vi "Test Sweep Manager.vi"(8 "error in (no error)":errorcluster, 11 "Lockin.DAQ in":refnum<class "Instrument.DAQ.lvclass">) -> (0 "error out":errorcluster, 3 "Lockin.DAQ out":refnum<class "Instrument.DAQ.lvclass">)   [LabVIEW 2019, in "Instrument.Lockin.lvlib" / "Instrument.DAQ.lvclass"]
uses:
  Instrument.DAQ.lvclass
  Typedefs/AO.Channel--Cluster--Array.ctl
  Typedefs/AO.Channel--Cluster.ctl
  Typedefs/AO.Channel.Function--Enum.ctl
  Typedefs/DAQ.Sampling.Sampling--Cluster.ctl
  Typedefs/Sweep.Configuration--Cluster.ctl
  Typedefs/Sweep.Channel--Cluster--Array.ctl
  Typedefs/Sweep.Channel--Cluster.ctl
  Typedefs/Sweep.Pattern--Enum.ctl
  Instrument.DAQ.lvclass/Instrument.DAQ.ctl
  <vilib>/Analysis/2dsp.llb/Decimate (single shot, DBL).vi
  <vilib>/Analysis/NI_AALPro.lvlib
  Instrument.Lockin/Instrument.Lockin.lvclass
panel:
  out "Waveform Graph 2":dbl[][](graph)
  in  "Sweep Pattern":cluster{"Channel":u16, "Sweep Pattern":dbl[]}[](array[cluster])=[{"Channel"=0, "Sweep Pattern"=[]}] {"Sweep Pattern" format="%#_3p"; "Channel" min=1 max=128}
  in  "milliseconds to wait":u32=1000
  out "Updates":i32
  out "Update":i32
  out "Waveform Graph":waveform(dbl)[](graph)
  in  "Configuration.Sweep":T1 {"Channels"."Table" format="%#_1f"; "Channels"."Channel" min=1 max=128; "Channels"."Start" format="%#_6p"; "Channels"."End" format="%#_6p"}
  in  "sampling":T5={"Fs"=204789.0, "#s"=15753} {"Fs" format="%#_13g"}
  in  "stop":bool
  in  "AO Channels":T6=[{"Enable?"=FALSE, "Channel"=0, "Amplitude"=0.0, "Offset"=0.0, "Frequency"=0.1, "Phase"=0.0, "Function"=enum."Sine", "Sweeping?"=FALSE}] {"Phase" format="%.3g"; "Frequency" min=0.0001 max=10000.0 format="%.3g"; "Offset" format="%.3p"; "Amplitude" min=0.0 max=10.0 format="%.3p"}
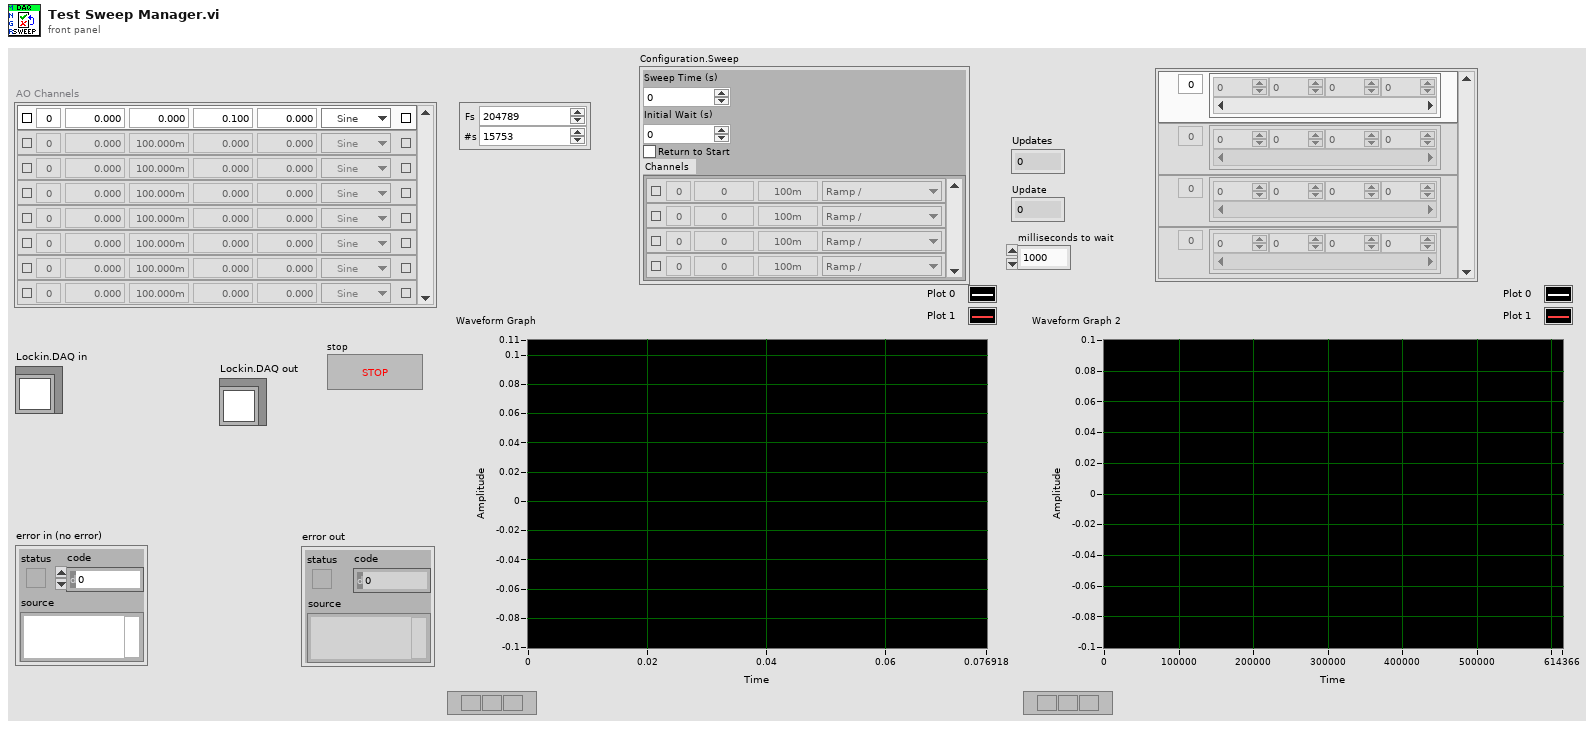
[diagram p1: front panel]
types:
  T1 = typedef "Instrument.Lockin.lvlib/Instrument.DAQ.lvclass/Sweep.Configuration--Cluster.ctl" = cluster{"Sweep Time (s)":dbl, "Initial Wait (s)":dbl, "Return to Start":bool, "Channels":T2}
  T2 = typedef "Instrument.Lockin.lvlib/Instrument.DAQ.lvclass/Sweep.Channel--Cluster--Array.ctl" = T3[]
  T3 = typedef "Instrument.Lockin.lvlib/Instrument.DAQ.lvclass/Sweep.Channel--Cluster.ctl" = cluster{"Enable?":bool, "Channel":u16, "Start":dbl, "End":dbl, "Pattern":T4, "Table":dbl[]}
  T4 = typedef "Instrument.Lockin.lvlib/Instrument.DAQ.lvclass/Sweep.Pattern--Enum.ctl" = enum16{"Ramp /", "Ramp /\\", "Smooth Ramp _/", "Smooth Ramp _/\\_", "Table"}
  T5 = typedef "Instrument.Lockin.lvlib/Instrument.DAQ.lvclass/DAQ.Sampling.Sampling--Cluster.ctl" = cluster{"Fs":dbl, "#s":i32}
  T6 = typedef "Instrument.Lockin.lvlib/Instrument.DAQ.lvclass/AO.Channel--Cluster--Array.ctl" = T7[]
  T7 = typedef "Instrument.Lockin.lvlib/Instrument.DAQ.lvclass/AO.Channel--Cluster.ctl" = cluster{"Enable?":bool, "Channel":i32, "Amplitude":dbl, "Offset":dbl, "Frequency":dbl, "Phase":dbl, "Function":T8, "Sweeping?":bool}
  T8 = typedef "Instrument.Lockin.lvlib/Instrument.DAQ.lvclass/AO.Channel.Function--Enum.ctl" = enum16{"Sine", "Triangle", "Square"}
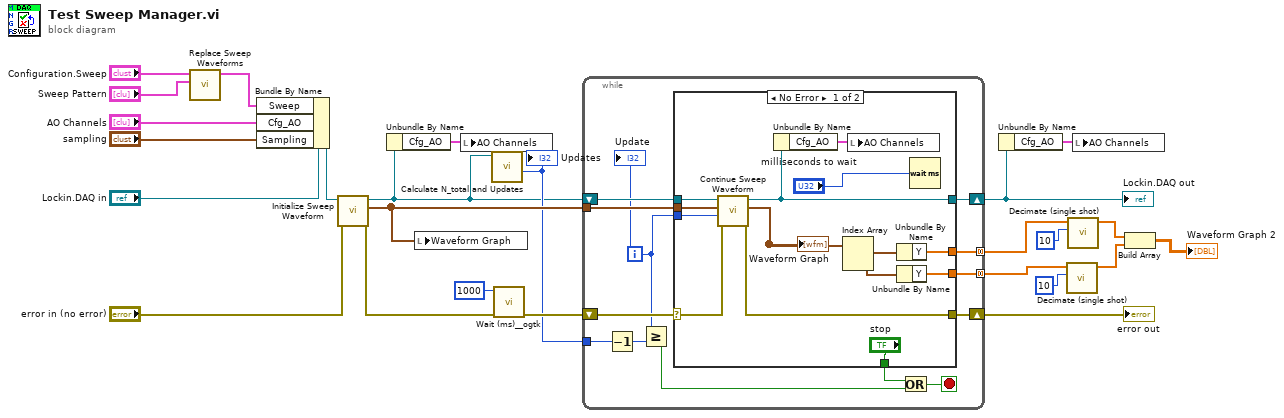
[diagram p0: block diagram]
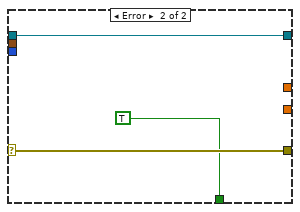
[diagram p2: hidden frame]
diagram:
  n1 = call "Replace Sweep Waveforms.vi"("Channels New"="Sweep Pattern", "Sweep in"="Configuration.Sweep") -> ("Sweep out"=w11:T1)  [unwired: 9 in]
  n2 = Bundle By Name(cluster="Lockin.DAQ in", "Sweep"=w11, "Cfg_AO"="AO Channels", "Sampling"="sampling") -> (w20:refnum<class "Instrument.DAQ.lvclass">)
  n3 = call "Initialize Sweep Waveform.vi"("error in (no error)"="error in (no error)", "Instrument.DAQ in"=w20) -> ("error out"=w15:errorcluster, "Waveforms"=w19:waveform(dbl)[], "Instrument.DAQ out"=w4:refnum<class "Instrument.DAQ.lvclass">)  [unwired: 7 in]
  n4 = Unbundle By Name(w4) -> ("Cfg_AO"=w3:T6)
  n5 = local write "Waveform Graph"(w19) -> ()
  n6 = local write "AO Channels"(w3) -> ()
  n7 = call "Calculate N_total and Updates.vi"("Instrument.DAQ in"=w4) -> ("Updates"=w16:i32)  [unwired: 8 in, 2 out]
  "Updates" <- w16
  n8 = call <userlib>:"Wait (ms)__ogtk.vi"("error in (no error)"=w15, "milliseconds to wait"=u32 1000) -> ("error out"=w18:errorcluster)  [unwired: 8 in, 1 out]
  n9 = while {
    shift-right: [w37] -> w25
    shift-left: w18 -> [w38]
    shift-right: [w35] -> w1
    shift-left: w4 -> [w36]
    tunnel: w19 -> [w34]
    tunnel: w16 -> [w32]
    tunnel: [w27] -> w14 mode=concatenating
    tunnel: [w26] -> w8 mode=concatenating
    i -> [w33]
    stop <- w29 stop-if-true
    n10 = Decrement(x=w32) -> (x-1=w28:i32)
    n11 = Greater Or Equal?(x=w33, y=w28) -> (x >= y?=w31:bool)
    n12 = case shown="No Error" w38 {
      selector: w38 -> [w48 w55]
      tunnel: [w51 w55] -> w37
      tunnel: [w39 w54] -> w35
      tunnel: w36 -> [w49 w54]
      tunnel: ["stop" TRUE ("stop")] -> w30
      tunnel: w34 -> [w50 _]
      tunnel: w33 -> [w47 _]
      tunnel: [w43 _] -> w27
      tunnel: [w41 _] -> w26
      frame No Error {
        n13 = call "Continue Sweep Waveform.vi"("error in (no error)"=w48, "Sweep Index"=w47, "Waveforms in"=w50, "Instrument.DAQ in"=w49) -> ("error out"=w51:errorcluster, "Waveforms out"=w45:waveform(dbl)[], "Instrument.DAQ out"=w39:refnum<class "Instrument.DAQ.lvclass">)  [unwired: 5 in]
        "Waveform Graph" <- w45
        n14 = Unbundle By Name(w39) -> ("Cfg_AO"=w40:T6)
        n15 = Index Array(array=w45) -> (element #1=w44:waveform(dbl), element #2=w42:waveform(dbl))  [unwired: 2 in]
        n16 = local write "AO Channels"(w40) -> ()
        n17 = Unbundle By Name(w44) -> ("Y"=w43:dbl[])
        n18 = Unbundle By Name(w42) -> ("Y"=w41:dbl[])
        n19 = Wait (ms)(milliseconds to wait="milliseconds to wait") -> ()  [unwired: 1 out]
      }
      frame Error {
      }
    }
    n20 = Or(x=w30, y=w31) -> (x .or. y?=w29:bool)
    "Update" <- w33
  }
  "error out" <- w25
  "Lockin.DAQ out" <- w1
  n21 = Unbundle By Name(w1) -> ("Cfg_AO"=w2:T6)
  n22 = call-poly <vilib>:"Decimate (single shot).vi"("decimating factor"=10, "X"=w8) -> ("Decimated Array"=w7:dbl[])  [unwired: 8 in, 1 out]
  n23 = call-poly <vilib>:"Decimate (single shot).vi"("decimating factor"=10, "X"=w14) -> ("Decimated Array"=w6:dbl[])  [unwired: 8 in, 1 out]
  n24 = local write "AO Channels"(w2) -> ()
  n25 = Build Array(w6, w7) -> (→"Waveform Graph 2":dbl[][])
